vi "Time domain Rx to normalized FFT.vi"(7 "Normalize to TF":bool=TRUE, 10 "window":T1=1 items=["Rectangle"=0, "Hanning"=1, "Hamming"=2, "Blackman-Harris"=3, "Exact Blackman"=4, "Blackman"=5, "Flat Top"=6, "4 Term B-Harris "=7, "7 Term B-Harris"=8, "Low Sidelobe"=9, "Blackman Nuttall"=11, "Triangle"=30, "Bartlett-Hanning"=31, "Bohman"=32, "Parzen"=33, "Welch"=34, "Kaiser"=60, "Dolph-Chebyshev"=61, "Gaussian"=62], 11 "Spec Waveform Baseline Sub":waveform(dbl)={"t0"=timestamp(3728232981.5205336 s since 1904-01-01), "dt"=9.9999999999997e-07, "Y"=array[20000 elements], "attributes"=variant("NI_ChannelName"=variant(string "H1/ai7"), "NI_UnitDescription"=variant(string "Volts"))}) -> (0 "Rx FFT _NoCorrect":cluster{"f0":dbl, "df":dbl, "magnitude":dbl[]}(graph), 1 "Waveform Graph":cluster{"f0":dbl, "df":dbl, "magnitude":dbl[]}(graph), 2 "TF units from loaded file":string, 3 "TF Corr Rx FFT complex":T2)   [LabVIEW 2021]
uses:
  <vilib>/Analysis/4window.llb/windowTd.ctl
  <vilib>/measure/maspectr.llb/Power Spectrum and PSD Export Mode.ctl
  <vilib>/measure/maspectr.llb/FFT Spectrum (Mag-Phase) for 1 Chan.vi
  <vilib>/measure/maspectr.llb/FFT Power Spectrum and PSD for 1 Chan.vi
  MPS_Labview/MPS_global_variables.vi
  <vilib>/measure/NI_MAPro.lvlib
  <vilib>/Analysis/NI_AALPro.lvlib
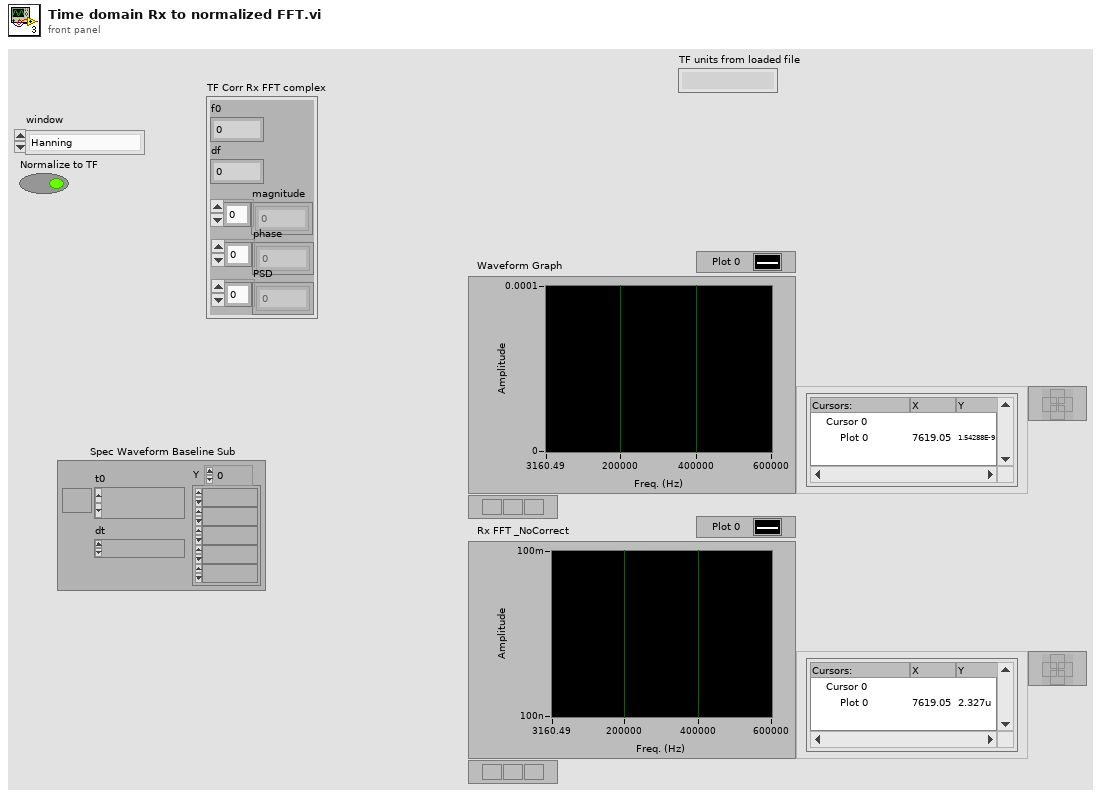
[diagram p1: front panel]
types:
  T1 = typedef "NI_AALPro.lvlib/windowTd.ctl" = u32
  T2 = cluster{"f0":dbl, "df":dbl, "magnitude":dbl[], "phase":dbl[], "PSD":dbl[]}
  T3 = typedef "NI_MAPro.lvlib/Power Spectrum and PSD Export Mode.ctl" = u16
  T4 = cluster{"f0":dbl, "df":dbl, "magnitude":dbl[], "phase":dbl[], dbl[]}
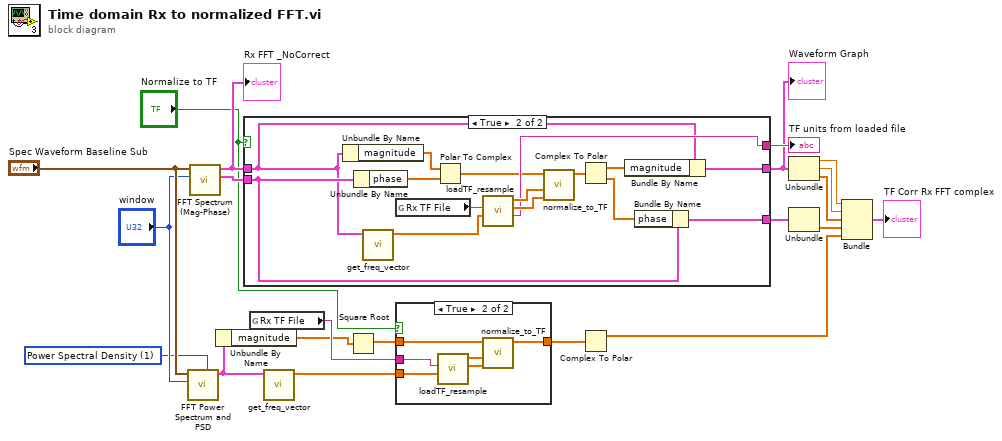
[diagram p0: block diagram]
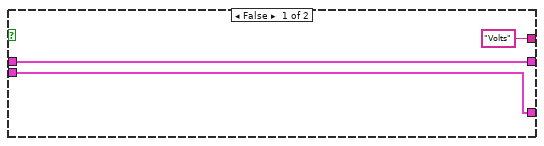
[diagram p3: hidden frame]
diagram:
  w4 = T3 1 items=["Power Spectrum", "Power Spectral Density"] ("export mode")
  n1 = call-poly <vilib>:"FFT Power Spectrum and PSD.vi"("export mode"=w4, "window"="window", "time signal"="Spec Waveform Baseline Sub") -> ("Power Spectrum / PSD"=w8:cluster{"f0":dbl, "df":dbl, "magnitude":dbl[]})  [unwired: 5 in, 3 out]
  n2 = call-poly <vilib>:"FFT Spectrum (Mag-Phase).vi"("window"="window", "time signal"="Spec Waveform Baseline Sub") -> ("phase"=w21:cluster{"f0":dbl, "df":dbl, "phase":dbl[]}, "magnitude"=w19:cluster{"f0":dbl, "df":dbl, "magnitude":dbl[]})  [unwired: 5 in, 3 out]
  "Rx FFT _NoCorrect" <- w19
  n3 = Unbundle By Name(w8) -> ("magnitude"=w1:dbl[])
  n4 = case shown="True" "Normalize to TF" {
    tunnel: w21 -> [w23 w34]
    tunnel: ["Volts" ("TF units from loaded file") w31] -> w20
    tunnel: w19 -> [w24 w25]
    tunnel: [w24 w27] -> w18
    tunnel: [w23 w26] -> w17
    frame False {
    }
    frame True {
      n5 = Unbundle By Name(w25) -> ("magnitude"=w36:dbl[])
      n6 = Unbundle By Name(w34) -> ("phase"=w35:dbl[])
      n7 = call "get_freq_vector.vi"("FFT magnitude"=w25) -> ("Freq array"=w37:dbl[])  [unwired: 10 in]
      n8 = global read "MPS_global_variables.vi" "Rx TF File"() -> (w32:string)
      n9 = Polar To Complex(1:w35, 2:w36) -> (0:w29:cdb[])
      n10 = call "loadTF_resample.vi"("desired freqs"=w37, "mat file name"=w32) -> ("TF units from loaded file"=w31:string, "output TF phase"=w39:dbl[], "output TF mag"=w38:dbl[])  [unwired: 7 in]
      n11 = call "normalize_to_TF.vi"("TF phase"=w39, "TF mag"=w38, "signal (can be complex)"=w29) -> ("signal normalized to TF (can be complex)"=w28:cdb[])  [unwired: 8 in]
      n12 = Complex To Polar(r * e^(i*theta)=w28) -> (r=w30:dbl[], theta=w33:dbl[])
      n13 = Bundle By Name(cluster=w25, "magnitude"=w30) -> (w27:cluster{"f0":dbl, "df":dbl, "magnitude":dbl[]})
      n14 = Bundle By Name(cluster=w34, "phase"=w33) -> (w26:cluster{"f0":dbl, "df":dbl, "phase":dbl[]})
    }
  }
  "TF units from loaded file" <- w20
  "Waveform Graph" <- w18
  n15 = global read "MPS_global_variables.vi" "Rx TF File"() -> (w10:string)
  n16 = call "get_freq_vector.vi"("FFT magnitude"=w8) -> ("Freq array"=w9:dbl[])  [unwired: 10 in]
  n17 = Square Root(x=w1) -> (sqrt(x)=w2:dbl[])
  n18 = case shown="True" "Normalize to TF" {
    tunnel: [w40 w46] -> w11
    tunnel: w10 -> [_ w45]
    tunnel: w9 -> [_ w44]
    tunnel: w2 -> [w40 w41]
    frame False {
    }
    frame True {
      n19 = call "loadTF_resample.vi"("desired freqs"=w44, "mat file name"=w45) -> ("output TF phase"=w42:dbl[], "output TF mag"=w43:dbl[])  [unwired: 7 in, 1 out]
      n20 = call "normalize_to_TF.vi"("TF phase"=w42, "TF mag"=w43, "signal (can be complex)"=w41) -> ("signal normalized to TF (can be complex)"=w46:cdb[])  [unwired: 8 in]
    }
  }
  n21 = Complex To Polar(r * e^(i*theta)=w11) -> (r=w7:dbl[])  [unwired: 1 out]
  n22 = Unbundle(w18) -> ("f0"=w16:dbl, "df"=w15:dbl, "magnitude"=w14:dbl[])
  n23 = Unbundle(w17) -> ("phase"=w13:dbl[])  [unwired: 2 out]
  n24 = Bundle("f0"=w16, "df"=w15, "magnitude"=w14, "phase"=w13, w7) -> (→"TF Corr Rx FFT complex":T4)  [unwired: 1 in]
